vi "Unflatten from YAML.vi"(8 "error in (no error)":errorcluster, 11 "YAML String":string) -> (0 "error out":errorcluster, 2 "Remaining String":string, 3 "Anything":variant)   [LabVIEW 2015, in "YAML Parser.lvlib"]
uses:
  YAML Parser.lvlib
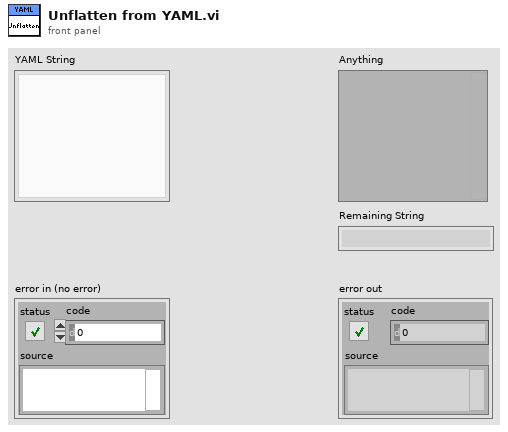
[diagram p1: front panel]
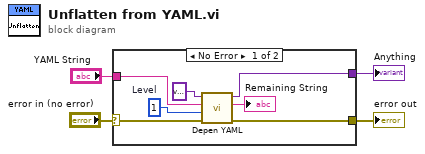
[diagram p0: block diagram]
diagram:
  n1 = case shown="No Error" "error in (no error)" {
    selector: "error in (no error)" -> [w11 w12]
    tunnel: [w8 w12] -> w3
    tunnel: "YAML String" -> [w10 _]
    tunnel: [w9 _] -> w1
    frame No Error {
      w6 = u32 1  # Level
      n2 = call "Depen YAML.vi"("error in (no error)"=w11, "Level"=w6, "YAML String"=w10, "Data in"=variant) -> ("error out"=w8:errorcluster, "Remaining String"=→"Remaining String":string, "Data out"=w9:variant)  [unwired: 5 in]
    }
    frame Error {
    }
  }
  "error out" <- w3
  "Anything" <- w1
